vi "Confirm Cycle Test.vi"(0 "GEA2 Reference In":refnum<k24>, 5 "Standalone?":bool, 7 "Enum":T1(ring), 11 "Error In":errorcluster) -> (4 "GEA2 Reference Out":refnum<k24>, 6 "Pass/Fail?":bool, 15 "Error Out":errorcluster)   [LabVIEW 2016, in "Centauro.lvlib"]
uses:
  Projects/Centauro.lvlib
  Q:/Common/DLLs/GEA3/GeaCommunication.dll
  Common/DLLs/GEA3/GeaCommunication.dll
  Common/LabVIEW GEA2 Toolkit/LabVIEW_GEA2_Toolkit.lvlibp/type defs/Source_Destination.ctl
  Common/LabVIEW GEA2 Toolkit/LabVIEW_GEA2_Toolkit.lvlibp/type defs/ERD Read Data In.ctl
  Common/LabVIEW GEA2 Toolkit/LabVIEW_GEA2_Toolkit.lvlibp/type defs/Data Type.ctl
  Common/LabVIEW GEA2 Toolkit/LabVIEW_GEA2_Toolkit.lvlibp
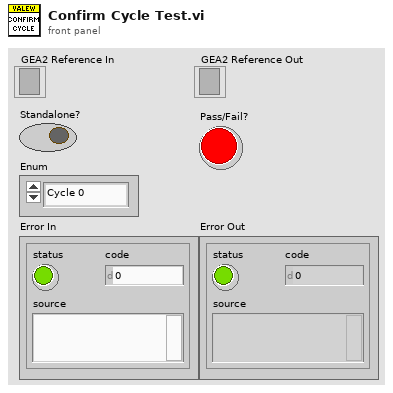
[diagram p1: front panel]
types:
  T1 = enum16{"Cycle 0", "Cycle 1", "Cycle 2", "Cycle 3", "Cycle 4", "Cycle 5", "Cycle 6", "Cycle 7", "Cycle 8", "Cycle 9", "Cycle 10", "Cycle 11", "Cycle 12", "Cycle 13"}
  T2 = typedef "LabVIEW_GEA2_Toolkit.lvlibp/ERD Read Data In.ctl" = cluster{"ERD Number":u16, "Data Type":T3}
  T3 = typedef "LabVIEW_GEA2_Toolkit.lvlibp/Data Type.ctl" = enum16{"string", "boolean", "uint8_t", "uint16_t", "uint32_t", "uint64_t", "int8_t", "int16_t", "int32_t", "int64_t"}
  T4 = typedef "LabVIEW_GEA2_Toolkit.lvlibp/Source_Destination.ctl" = cluster{"Source":u8, "Destination":u8}
  T5 = typedef "LabVIEW_GEA2_Toolkit.lvlibp/ERD Read Data Out.ctl" = cluster{"ERD Number":u16, "Data":string}
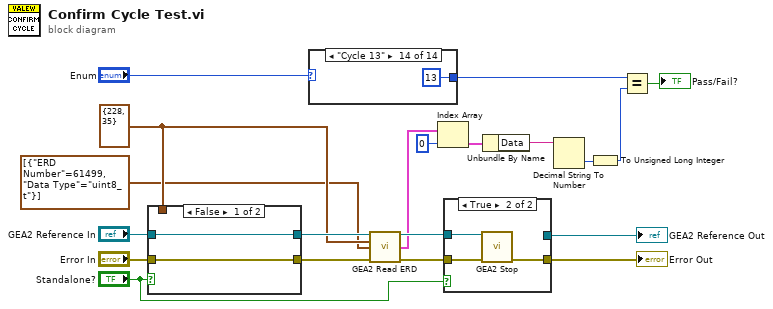
[diagram p0: block diagram]
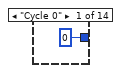
[diagram p2: hidden frame]
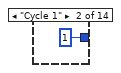
[diagram p3: hidden frame]
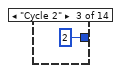
[diagram p4: hidden frame]
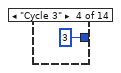
[diagram p5: hidden frame]
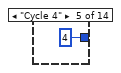
[diagram p6: hidden frame]
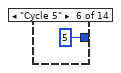
[diagram p7: hidden frame]
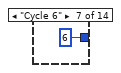
[diagram p8: hidden frame]
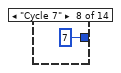
[diagram p9: hidden frame]
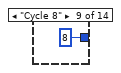
[diagram p10: hidden frame]
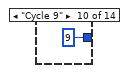
[diagram p11: hidden frame]
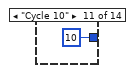
[diagram p12: hidden frame]
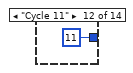
[diagram p13: hidden frame]
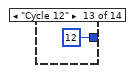
[diagram p14: hidden frame]
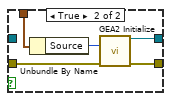
[diagram p16: hidden frame]
diagram:
  w12 = T4 {"Source"=228, "Destination"=35} ("GEA Inputs")
  n1 = case shown="False" "Standalone?" {
    tunnel: "Error In" -> [w21 w27]
    tunnel: [w21 w26] -> w16
    tunnel: "GEA2 Reference In" -> [w22 _]
    tunnel: [w22 w25] -> w14
    tunnel: w12 -> [_ w23]
    frame False {
    }
    frame True {
      n2 = Unbundle By Name(w23) -> ("Source"=w24:u8)
      n3 = call "GEA2 Initialize.vi"("Source Address"=w24, "error in"=w27) -> ("GEA2 Reference Out"=w25:refnum<k24>, "error out"=w26:errorcluster)  [unwired: 11 in, 1 out]
    }
  }
  n4 = case shown="\"Cycle 13\"" "Enum" {
    tunnel: [u32 0 u32 1 u32 2 u32 3 u32 4 u32 5 u32 6 u32 7 u32 8 u32 9 u32 10 u32 11 u32 12 u32 13] -> w4
    frame "Cycle 0" {
    }
    frame "Cycle 1" {
    }
    frame "Cycle 2" {
    }
    frame "Cycle 3" {
    }
    frame "Cycle 4" {
    }
    frame "Cycle 5" {
    }
    frame "Cycle 6" {
    }
    frame "Cycle 7" {
    }
    frame "Cycle 8" {
    }
    frame "Cycle 9" {
    }
    frame "Cycle 10" {
    }
    frame "Cycle 11" {
    }
    frame "Cycle 12" {
    }
    frame "Cycle 13" {
    }
  }
  n5 = call "GEA2 Read ERD.vi"("GEA2 Reference In"=w14, "GEA Inputs"=w12, "Read ERD List"=T2[] [{"ERD Number"=61499, "Data Type"=enum."uint8_t"}], "Error In"=w16) -> ("GEA2 Reference Out"=w13:refnum<k24>, "ERD Data Out"=w10:T5[], "Error Out"=w15:errorcluster)  [unwired: 8 in, 1 out]
  n6 = Index Array(array=w10, index=0) -> (element=w8:T5)
  n7 = case shown="True" "Standalone?" {
    tunnel: [w43 w46] -> w18
    tunnel: w15 -> [w43 w45]
    tunnel: w13 -> [w42 w44]
    tunnel: [w42 _] -> w1
    frame False {
    }
    frame True {
      n8 = call "GEA2 Stop.vi"("GEA2 Reference In"=w44, "Error In"=w45) -> ("Error Out"=w46:errorcluster)  [unwired: 13 in]
    }
  }
  "Error Out" <- w18
  "GEA2 Reference Out" <- w1
  n9 = Unbundle By Name(w8) -> ("Data"=w7:string)
  n10 = Decimal String To Number(string=w7) -> (number=w3:i32)  [unwired: 2 in, 1 out]
  n11 = To Unsigned Long Integer(number=w3) -> (unsigned 32bit integer=w2:u32)
  n12 = Equal?(x=w4, y=w2) -> (x = y?=→"Pass/Fail?":bool)
